vi "Test.vi"() -> ()   [LabVIEW 2015]
uses:
  Filter Data.ctl
  Filter XCtl.xctl
panel:
  in  "Exit":bool
  in  "Apply":bool
  in  "Filter XCtl":T1(xcontrol)
  out "Filter out":T2 {"IIR Filter Cluster"."Forward Coefficients" format="%.4f"; "IIR Filter Cluster"."Reverse Coefficients" format="%.4f"}
  in  "Filter":T2 {"IIR Filter Cluster"."Forward Coefficients" format="%.4f"; "IIR Filter Cluster"."Reverse Coefficients" format="%.4f"}
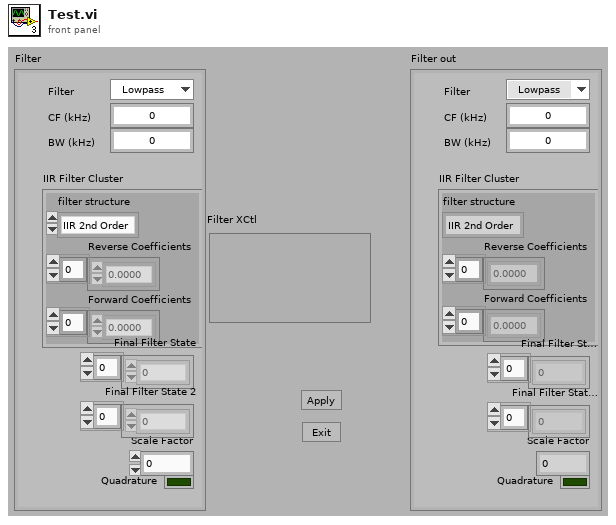
[diagram p1: front panel]
types:
  T1 = cluster{"CF (kHz)":dbl, "BW (kHz)":dbl, "IIR Filter Cluster":cluster{"filter structure":enum32{"IIR 2nd Order", "IIR 4th Order"}, "Reverse Coefficients":dbl[], "Forward Coefficients":dbl[]}, "Final Filter State":dbl[], "Scale Factor":dbl, "Final Filter State 2":dbl[], "Quadrature":bool, "Type":enum16{"Lowpass", "Highpass", "Bandpass", "Bandstop", "OFF"}}
  T2 = typedef "Filter XCtl.xctl/Filter Data.ctl" = cluster{"CF (kHz)":dbl, "BW (kHz)":dbl, "IIR Filter Cluster":cluster{"filter structure":enum32{"IIR 2nd Order", "IIR 4th Order"}, "Reverse Coefficients":dbl[], "Forward Coefficients":dbl[]}, "Final Filter State":dbl[], "Scale Factor":dbl, "Final Filter State 2":dbl[], "Quadrature":bool, "Type":enum16{"Lowpass", "Highpass", "Bandpass", "Bandstop", "OFF"}}
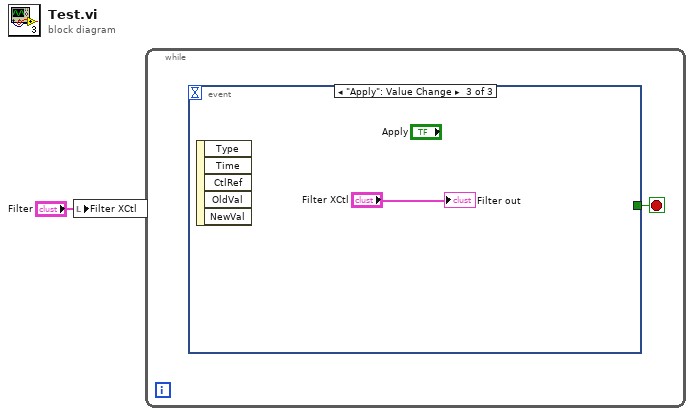
[diagram p0: block diagram]
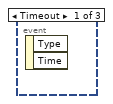
[diagram p2: hidden frame]
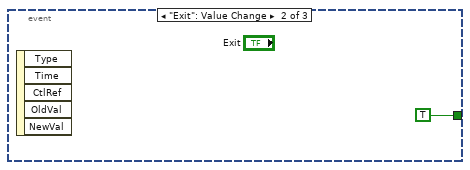
[diagram p3: hidden frame]
diagram:
  n1 = local write "Filter XCtl"("Filter") -> ()
  n2 = while {
    stop <- w2 stop-if-true
    n3 = event shown="[2] \"Apply\": Value Change" {
      selector: _ -> [_ _ _]
      dyn-events: _ -> [_ _ _]
      timeout: _ -> [_ _ _]
      tunnel: [_ TRUE _] -> w2
      event Timeout {
        n4 = event-data() -> ()  [unwired: 1 in, 2 out]
      }
      event "Exit": Value Change {
        n5 = event-data() -> ()  [unwired: 1 in, 5 out]
      }
      event "Apply": Value Change {
        n6 = event-data() -> ()  [unwired: 1 in, 5 out]
        "Filter out" <- "Filter XCtl"
      }
    }
  }
